vi "Evaluar.vi"(8 "error in (no error)":errorcluster, 11 "Prueba21_1 in":refnum<class "Prueba21.lvclass">) -> (0 "error out":errorcluster, 2 "pasa?":bool, 3 "Prueba21_1 out":refnum<class "Prueba21.lvclass">)   [LabVIEW 2019, in "Prueba21.lvclass"]
uses:
  Prueba21.lvclass
  Prueba21.lvclass/Prueba21.ctl
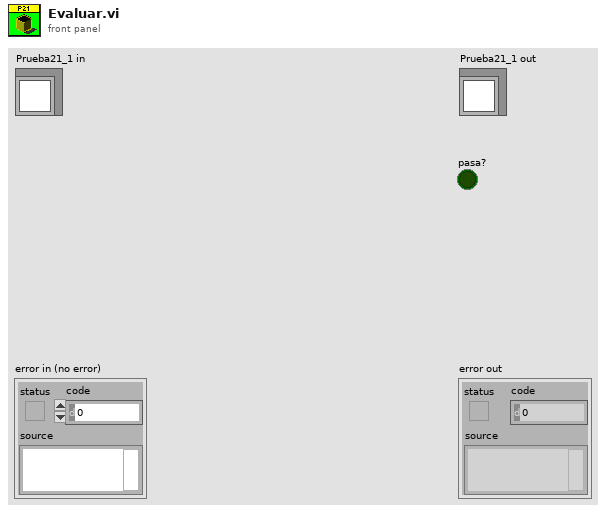
[diagram p1: front panel]
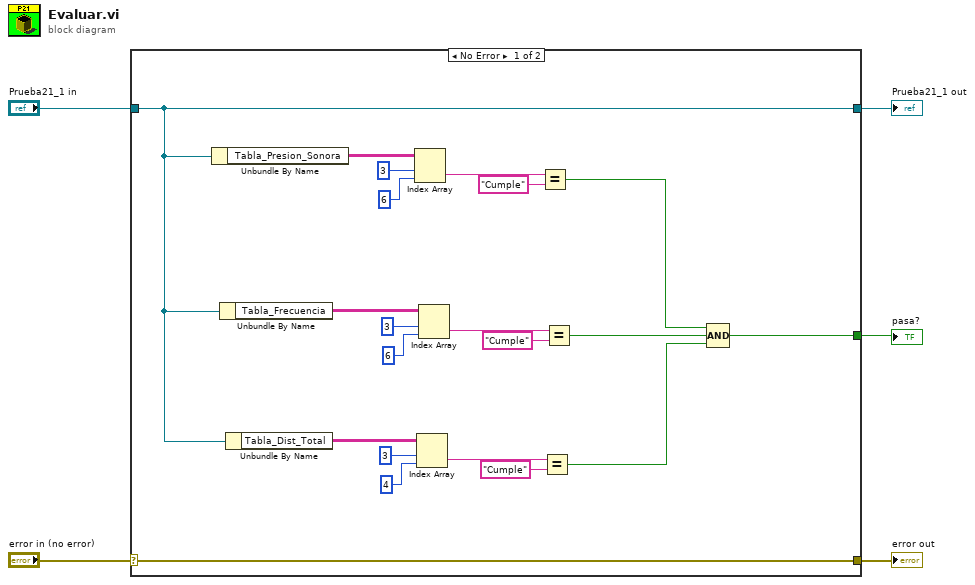
[diagram p0: block diagram]
diagram:
  n1 = case shown="No Error" "error in (no error)" {
    selector: "error in (no error)" -> [w26 w28]
    tunnel: [w26 w28] -> w4
    tunnel: [w25 w27] -> w2
    tunnel: "Prueba21_1 in" -> [w25 w27]
    tunnel: [w22 _] -> w1
    frame No Error {
      n2 = Unbundle By Name(w25) -> ("Tabla_Presion_Sonora"=w24:string[][])
      n3 = Unbundle By Name(w25) -> ("Tabla_Frecuencia"=w12:string[][])
      n4 = Unbundle By Name(w25) -> ("Tabla_Dist_Total"=w11:string[][])
      n5 = Index Array(array=w24, index (row)=3 ("disabled index (row)"), index (col)=6 ("disabled index (col)")) -> (element=w20:string)
      n6 = Index Array(array=w11, index (row)=3 ("disabled index (row)"), index (col)=4 ("disabled index (col)")) -> (element=w9:string)
      n7 = Index Array(array=w12, index (row)=3 ("disabled index (row)"), index (col)=6 ("disabled index (col)")) -> (element=w10:string)
      n8 = Equal?(x=w20, y="Cumple") -> (x = y?=w8:bool)
      n9 = Equal?(x=w9, y="Cumple") -> (x = y?=w6:bool)
      n10 = Equal?(x=w10, y="Cumple") -> (x = y?=w7:bool)
      n11 = Compound Arithmetic op=AND(w8, w7, w6) -> (w22:bool)
    }
    frame Error {
    }
  }
  "error out" <- w4
  "Prueba21_1 out" <- w2
  "pasa?" <- w1
